vi "CoinFlip.vi"() -> ()   [LabVIEW 2019]
uses:
  <vilib>/Analysis/6fits.llb/Curve Fitting Criteria.ctl
  <vilib>/numeric/Random Number (Range) U64.vi
  <vilib>/numeric/sub_Random U32.vi
  <vilib>/Analysis/NI_AALPro.lvlib
panel:
  out "mean squared error":dbl
  out "Coefficients polynomial fit":dbl[](array[numeric])
  out "weighted mean square error":dbl
  out "intercept":dbl
  out "slope":dbl
  out "Probability":dbl
  out "?":dbl[][](graph)
  in  "Amount":i32
  # "0 = heads\n1 = tails"
  # "Lineair model =>"
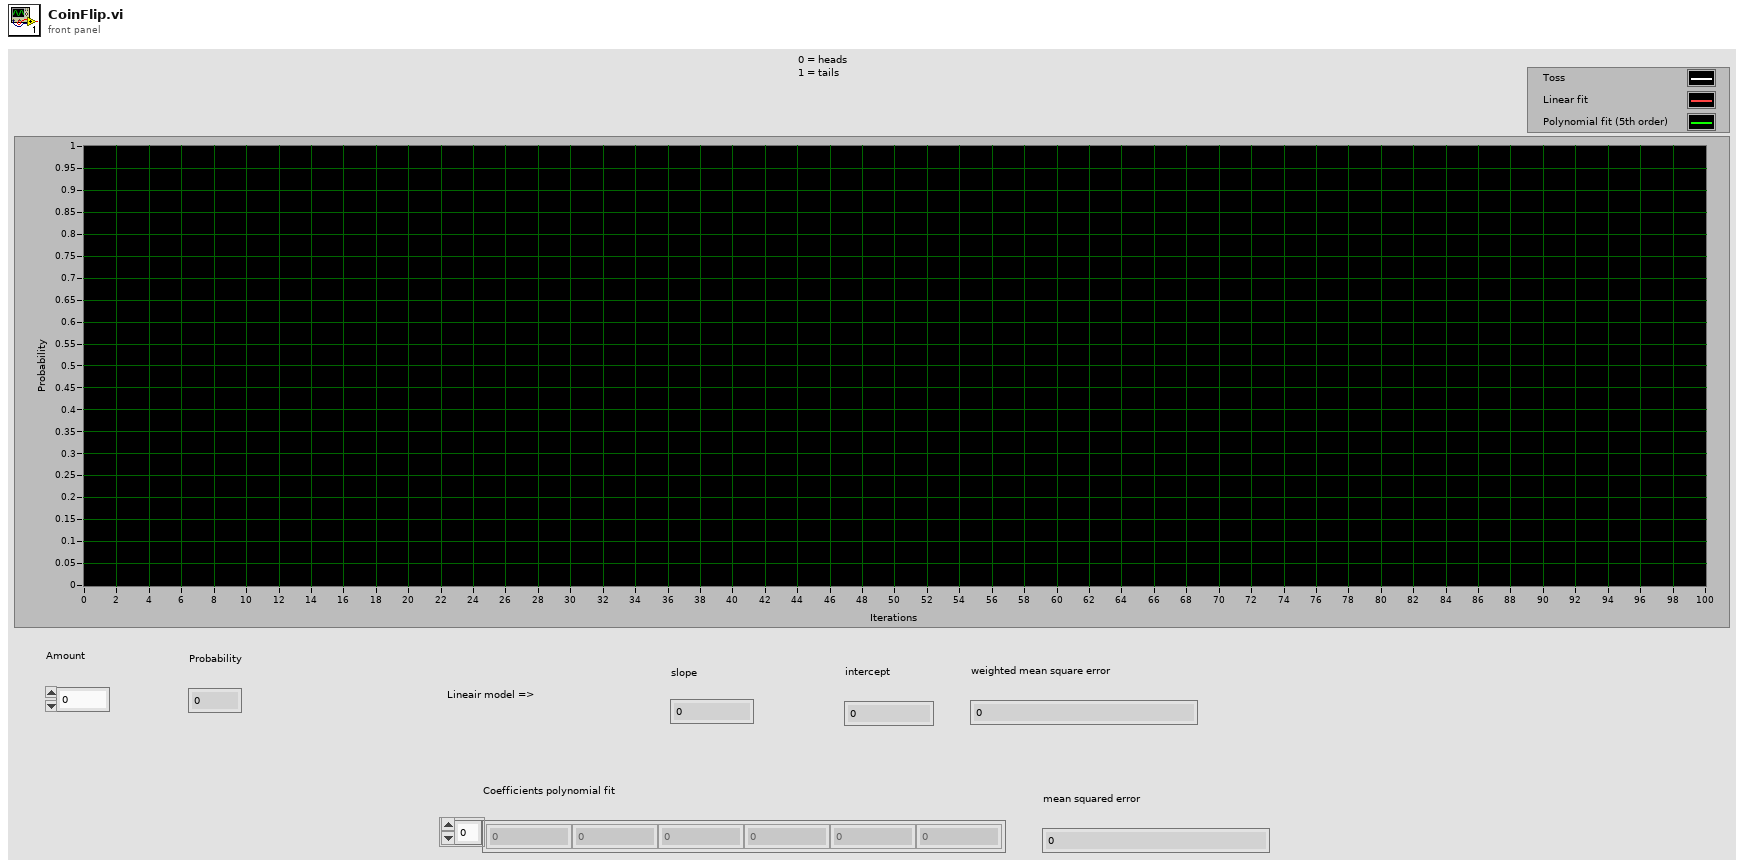
[diagram p1: front panel]
types:
  T1 = typedef "NI_AALPro.lvlib/Curve Fitting Criteria.ctl" = u16
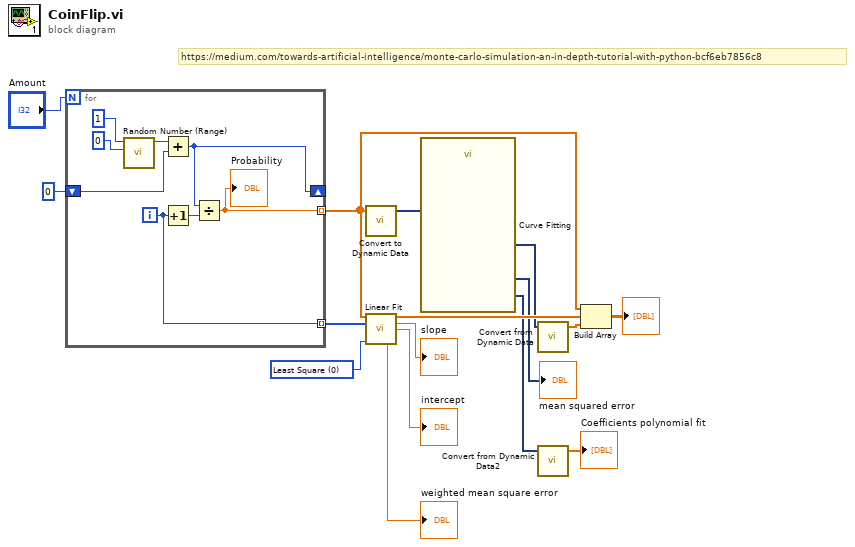
[diagram p0: block diagram]
diagram:
  w1 = T1 0 items=["Least Square", "Least Absolute Residual", "Bisquare"] ("method")
  # "https://medium.com/towards-artificial-intelligence/monte-carlo-simulation-an-in-depth-tutorial-with-python-bcf6eb7856c8"
  n1 = for {
    N: "Amount" -> [_]
    shift-right: [w20] -> _
    shift-left: u64 0 -> [w21]
    tunnel: [w18] -> w11 mode=indexing
    tunnel: [w17] -> w14 mode=indexing
    i -> [w17]
    n2 = call-poly <vilib>:"Random Number (Range).vi"("lower bound (0)"=u64 0, "upper bound (100)"=u64 1) -> ("number"=w22:u64)  [unwired: 9 in]
    n3 = Add(x=w22, y=w21) -> (x+y=w20:u64)
    n4 = Increment(x=w17) -> (x+1=w19:i32)
    n5 = Divide(x=w20, y=w19) -> (x/y=w18:dbl)
    "Probability" <- w18
  }
  n6 = call "Convert to Dynamic Data"("Array"=w11) -> ("Dynamic Data Type"=w10:dynamicdata)  [unwired: 3 in]
  n7 = call <vilib>:"Linear Fit.vi"("Y"=w11, "X"=w14, "method"=w1) -> ("Best Linear Fit"=w13:dbl[], "slope"=→"slope":dbl, "intercept"=→"intercept":dbl, "residue"=→"weighted mean square error":dbl)  [unwired: 8 in, 1 out]
  n8 = call "Curve Fitting"("Signals"=w10) -> ("mean squared error"=→"mean squared error":dynamicdata, "best fit"=w9:dynamicdata, "polynomial coefficients"=w7:dynamicdata)  [unwired: 6 in, 2 out]
  n9 = call "Convert from Dynamic Data"("Dynamic Data Type"=w9) -> ("Array"=w8:dbl[])  [unwired: 3 in]
  n10 = call "Convert from Dynamic Data2"("Dynamic Data Type"=w7) -> ("Array"=→"Coefficients polynomial fit":dbl[])  [unwired: 3 in]
  n11 = Build Array(w11, w13, w8) -> (→"?":dbl[][])
